vi "LVClass_CorrectionDataManager Compute_SlopesFromPositions.vi"(0 "CorrectionDataManager in":refnum<class "CorrectionDataManager.lvclass">, 5 "position":sgl[](array[numeric]), 7 "HasoSlopes in":refnum<class "HasoSlopes.lvclass">, 11 "error in (no error)":errorcluster) -> (4 "CorrectionDataManager out":refnum<class "CorrectionDataManager.lvclass">, 8 "HasoSlopes out":refnum<class "HasoSlopes.lvclass">, 15 "error out":errorcluster)   [LabVIEW 2020, in "CorrectionDataManager.lvclass"]
doc: "Simulation of the expected slopes given a wavefront corrector command.\n\n<B>corrdata_managerIn</B> : CorrDataManager object.\n<B>corrdata_managerOut</B> : CorrDataManager object.\n<B>command</B> : Array of size actuators count, containing for each actuator its current\n position.\n<B>HasoSlopes</B> : HasoSlopes object, where the simulated slopes are stored."
uses:
  CorrectionDataManager.lvclass
  HasoSlopes.lvclass
  CorrectionDataManager.lvclass/CorrectionDataManager.ctl
  LVClass_HasoSlopes Read HasoSlopes _ property.vi
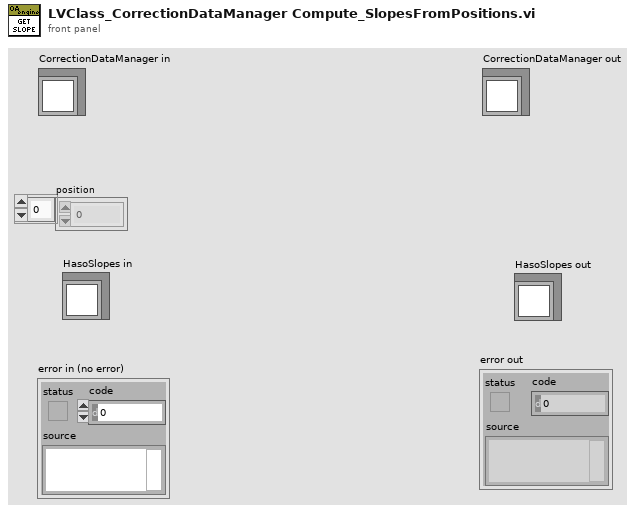
[diagram p1: front panel]
types:
  T1 = typedef "ClassID.ctl" = i64
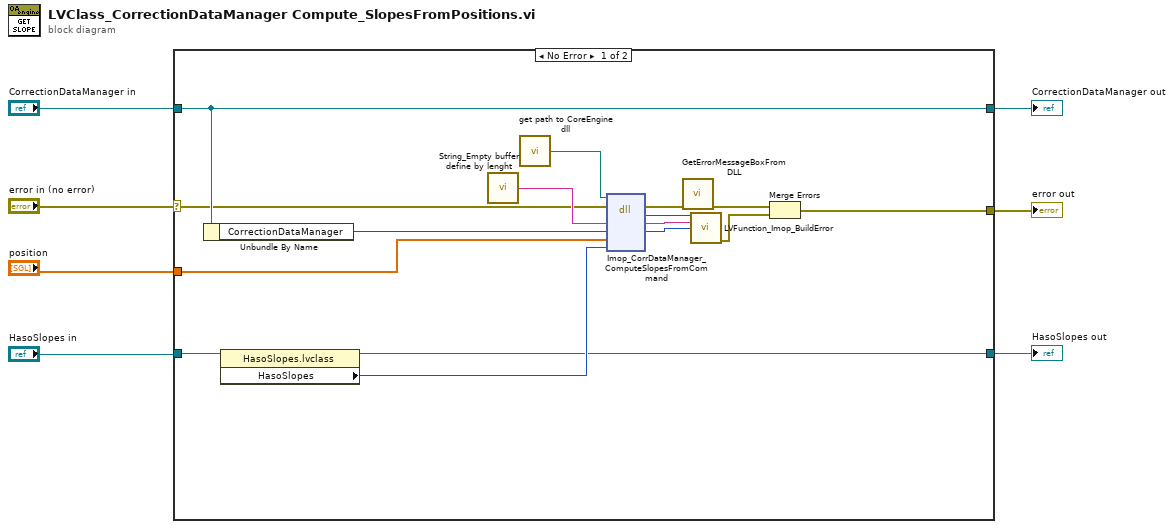
[diagram p0: block diagram]
diagram:
  n1 = case shown="No Error" "error in (no error)" {
    selector: "error in (no error)" -> [w11 w26]
    tunnel: [w21 w26] -> w5
    tunnel: [w20 w25] -> w4
    tunnel: "CorrectionDataManager in" -> [w20 w25]
    tunnel: "HasoSlopes in" -> [w13 w24]
    tunnel: [w10 w24] -> w2
    tunnel: "position" -> [w9 _]
    frame No Error {
      n2 = Unbundle By Name(w20) -> ("CorrectionDataManager"=w14:T1)
      n3 = property class="HasoSlopes.lvclass"(reference=w13) -> (reference out=w10:refnum<class "HasoSlopes.lvclass">, "HasoSlopes"=w12:T1)  [unwired: 1 in, 1 out]
      n4 = call "String_Empty buffer define by lenght.vi"() -> ("Empty buffer"=w18:string)  [unwired: 1 in]
      n5 = call "get path to CoreEngine dll.vi"() -> ("path to wavekit library"=w19:path)  [unwired: 14 in, 1 out]
      n6 = dll-call lib="D:/FLE/0.Code/CoreEngine4_Suite/LV2011_interface/DLLs/c_interface_vc100.dll" fn="Imop_CorrDataManager_ComputeSlopesFromCommand"(path in=w19, error in=w11, "message"=w18, "WavefrontCorrection"=w14, "position"=w9, "HasoSlopes"=w12) -> (error out=w17:errorcluster, "return type"=w16:i32, "message"=w15:string, "WavefrontCorrection"=w8:i64)  [unwired: 3 in, 1 out]
      n7 = call "GetErrorMessageBoxFromDLL.vi"("error IN"=w17) -> ("error OUT"=w23:errorcluster)  [unwired: 10 in]
      n8 = call "LVFunction_Imop_BuildError.vi"("code"=w16, "String to Prepend to source (\"\")"=w15, "Adresse"=w8) -> ("error out"=w22:errorcluster)  [unwired: 12 in]
      n9 = Merge Errors(w23, w22) -> (w21:errorcluster)
    }
    frame Error {
    }
  }
  "error out" <- w5
  "CorrectionDataManager out" <- w4
  "HasoSlopes out" <- w2
